vi "zc cleanup orphaned shm segments.vi"(8 "error in (no error)":errorcluster) -> (0 "error out":errorcluster)   [LabVIEW 2021, in "zenohc.lvlib"]
doc: "void zc_cleanup_orphaned_shm_segments(void);"
uses:
  zenohc.lvlib
  zenohc.dll
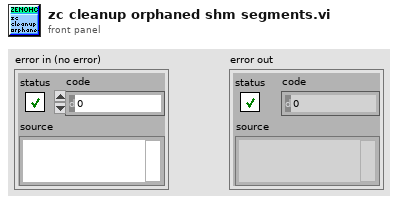
[diagram p1: front panel]
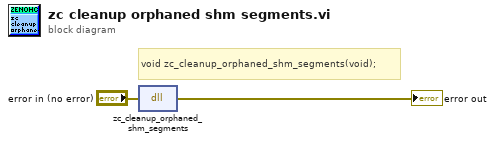
[diagram p0: block diagram]
diagram:
  # "void zc_cleanup_orphaned_shm_segments(void);"
  n1 = dll-call lib="D:/dev/zenoh_labview/zenohc/zenohc.*" fn="zc_cleanup_orphaned_shm_segments"(error in="error in (no error)") -> (error out=→"error out":errorcluster)  [unwired: 3 in, 1 out]
